vi "Update Header.vi"(8 "error in (no error)":errorcluster, 11 "CIFFIFO in":refnum<class "CIFfifo.lvclass">) -> (0 "error out":errorcluster, 3 "CIFFIFO out":refnum<class "CIFfifo.lvclass">)   [LabVIEW 2021, in "CIFfifo.lvclass"]
uses:
  CIFfifo.lvclass
  CIFfifo.lvclass/CIFfifo.ctl
  ChannelCommon/ChannelCommon.lvlib
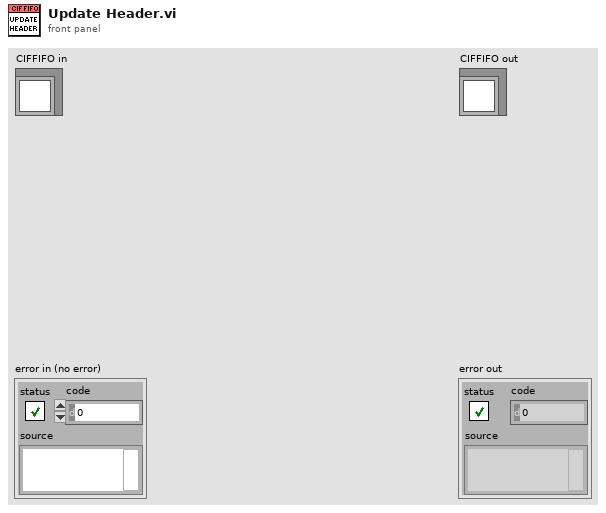
[diagram p1: front panel]
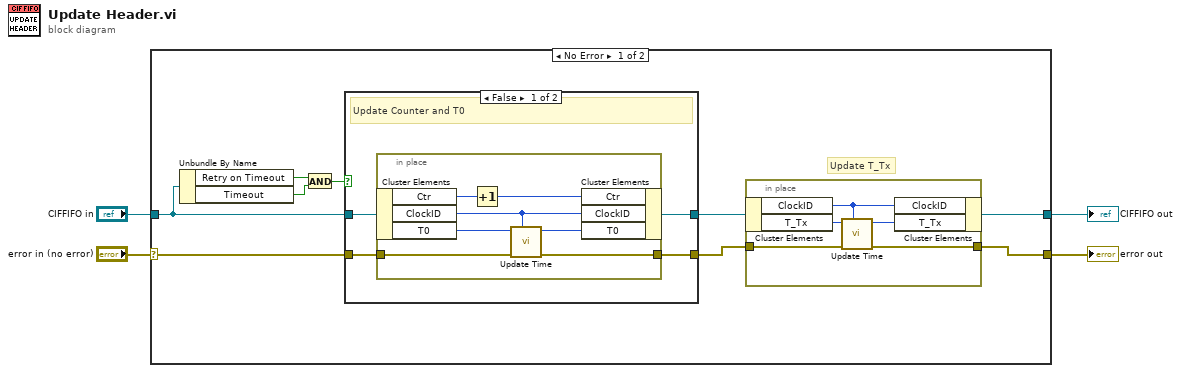
[diagram p0: block diagram]
diagram:
  n1 = case shown="No Error" "error in (no error)" {
    selector: "error in (no error)" -> [w6 w33]
    tunnel: [w11 w33] -> w3
    tunnel: [w10 w32] -> w1
    tunnel: "CIFFIFO in" -> [w13 w32]
    frame No Error {
      # "Update T_Tx"
      n2 = Unbundle By Name(w13) -> ("Retry on Timeout"=w9:bool, "Timeout"=w8:bool)
      n3 = And(x=w9, y=w8) -> (x .and. y?=w7:bool)
      n4 = case shown="False" w7 {
        tunnel: w13 -> [w22 w31]
        tunnel: [w20 w31] -> w12
        tunnel: w6 -> [w21 w30]
        tunnel: [w19 w30] -> w5
        frame False {
          # "Update Counter and T0"
          n5 = in-place {
            in-place-border: w21 -> [w24]
            in-place-border: [w23] -> w19
            n6 = in-place-cluster #1(w22) -> ("Ctr"=w29:u64, "ClockID"=w25:u8, "T0"=w27:u64)
            n7 = Increment(x=w29) -> (x+1=w28:u64)
            n8 = call "Update Time.vi"("ClockID"=w25, "error in (no error)"=w24, "Time in"=w27) -> ("error out"=w23:errorcluster, "Time out"=w26:u64)  [unwired: 7 in]
            n9 = in-place-cluster #1("Ctr"=w28, "ClockID"=w25, "T0"=w26) -> (w20:refnum<class "CIFfifo.lvclass">)
          }
        }
        frame True {
          # "Retry last packet"
        }
      }
      n10 = in-place {
        in-place-border: w5 -> [w16]
        in-place-border: [w15] -> w11
        n11 = in-place-cluster #2(w12) -> ("ClockID"=w14:u8, "T_Tx"=w18:u64)
        n12 = call "Update Time.vi"("ClockID"=w14, "error in (no error)"=w16, "Time in"=w18) -> ("error out"=w15:errorcluster, "Time out"=w17:u64)  [unwired: 7 in]
        n13 = in-place-cluster #2("ClockID"=w14, "T_Tx"=w17) -> (w10:refnum<class "CIFfifo.lvclass">)
      }
    }
    frame Error {
    }
  }
  "error out" <- w3
  "CIFFIFO out" <- w1
